vi "Init.vi"(8 "error in (no error)":errorcluster, 11 "Data in":refnum<class "Vector of Elements.lvclass">) -> (0 "error out":errorcluster, 3 "Data out":refnum<class "Vector of Elements.lvclass">)   [LabVIEW 2021, in "Vector of Elements.lvclass"]
uses:
  Vector of Elements.lvclass
  C:/Users/Tim/Documents/GitHub/LV_Abstract/Source/Element/Vector Parent/Vector Parent.lvclass
  Abs_Types/Type/Abs_Type.lvclass
  Element/Vector Parent/Vector Parent.lvclass/Vector Parent.ctl
  Vector of Elements.lvclass/Vector of Elements.ctl
  Element/Vector Parent/Properties/Read Size.vi
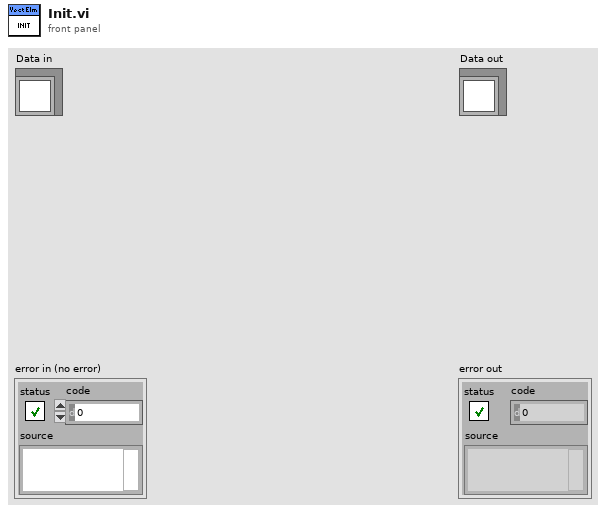
[diagram p1: front panel]
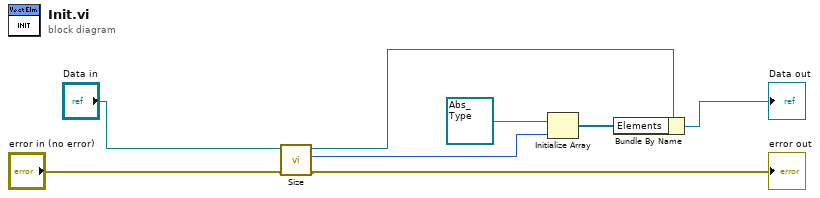
[diagram p0: block diagram]
diagram:
  n1 = call-dynamic "Size.vi"("error in (no error)"="error in (no error)", "Vector Parent in"="Data in") -> ("error out"=→"error out":errorcluster, "size"=w1:i32, "Vector Parent out"=w2:refnum<class "Vector of Elements.lvclass">)  [unwired: 7 in]
  n2 = Initialize Array(refnum<class "Abs_Type.lvclass"> refnum ("Element.lvlib:Element.lvclass"), w1) -> (w7:refnum<class "Abs_Type.lvclass">[])
  n3 = Bundle By Name(cluster=w2, "Elements"=w7) -> (→"Data out":refnum<class "Vector of Elements.lvclass">)
